vi "Global_Application Path.vi"(1 "Use ExeFilePath":bool) -> (0 "程序路径":path)   [LabVIEW 2011]
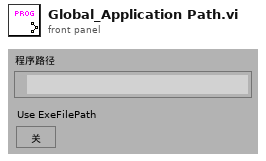
[diagram p1: front panel]
types:
  T1 = enum32{"invalid app kind", "Development System", "Run Time System", "Student Edition", "Embedded LabVIEW", "Evaluation", "Custom"}
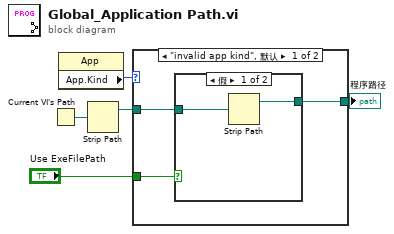
[diagram p0: block diagram]
diagram:
  n1 = Current VI's Path() -> (path=w5:path)
  n2 = property class="App"() -> ("App.Kind"=w4:T1)  [unwired: 2 in, 2 out]
  n3 = Strip Path(path=w5) -> (stripped path=w2:path)  [unwired: 1 out]
  n4 = case shown="\"invalid app kind\", 默认" w4 {
    tunnel: w2 -> [w8 w12]
    tunnel: [w7 w12] -> w3
    tunnel: "Use ExeFilePath" -> [w6 _]
    frame "invalid app kind", Default {
      n5 = case shown="假" w6 {
        tunnel: w8 -> [w10 w11]
        tunnel: [w9 w11] -> w7
        frame False {
          n6 = Strip Path(path=w10) -> (stripped path=w9:path)  [unwired: 1 out]
        }
        frame True {
        }
      }
    }
    frame "Development System" {
    }
  }
  "程序路径" <- w3
